vi "newValueStep.vi"(8 "error in (no error)":errorcluster, 11 "RampAction in":refnum<class "RampAction.lvclass">) -> (0 "error out":errorcluster, 3 "RampAction out":refnum<class "RampAction.lvclass">)   [LabVIEW 2009, in "Views.lvlib" / "ScriptEditor.lvlib" / "RampAction.lvclass"]
uses:
  RampAction.lvclass
  RampAction.lvclass/RampAction.ctl
  Tools/Scripting/ScriptingEvent/ScriptEvents/Ramp/RampEvent/RampEvent.lvclass
  ActionPanel.lvclass
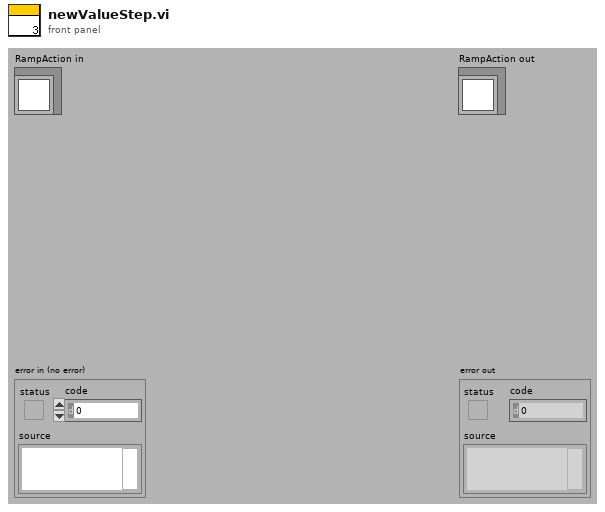
[diagram p1: front panel]
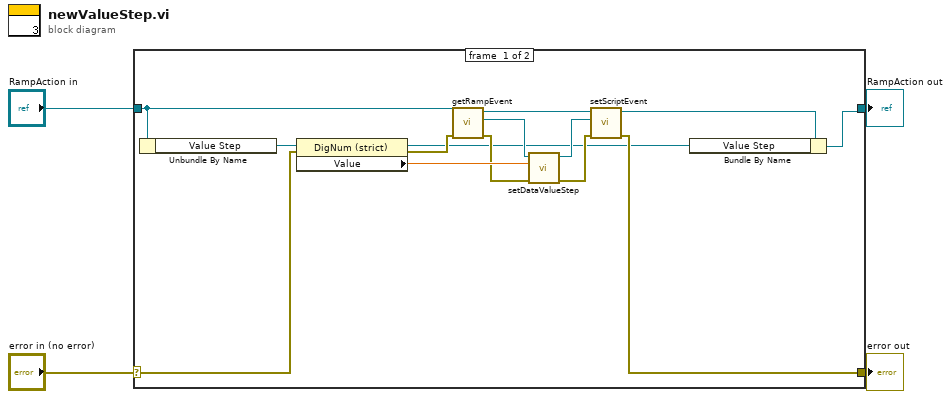
[diagram p0: block diagram]
diagram:
  n1 = case shown="No Error" "error in (no error)" {
    selector: "error in (no error)" -> [w17 w20]
    tunnel: [w8 w20] -> w3
    tunnel: [w5 w19] -> w1
    tunnel: "RampAction in" -> [w16 w19]
    frame #0 {
      n2 = Unbundle By Name(w16) -> ("Value Step"=w18:refnum<vi>)
      n3 = property class="DigNum (strict)"(reference=w18, error in=w17) -> (reference out=w7:refnum<vi>, error out=w15:errorcluster, "Value"=w13:dbl)
      n4 = call "getRampEvent.vi"("error in (no error)"=w15, "RampAction in"=w16) -> ("error out"=w12:errorcluster, "RampEvent"=w14:refnum<class "RampEvent.lvclass">, "RampAction out"=w11:refnum<class "RampAction.lvclass">)  [unwired: 7 in]
      n5 = call "setDataValueStep.vi"("error in (no error)"=w12, "dataValueStep"=w13, "RampEvent.lvclass in"=w14) -> ("error out"=w9:errorcluster, "RampEvent.lvclass out"=w10:refnum<class "RampEvent.lvclass">)  [unwired: 7 in]
      n6 = call "setScriptEvent.vi"("error in (no error)"=w9, "ScriptEvent.lvclass"=w10, "ActionPanel.lvclass in"=w11) -> ("error out"=w8:errorcluster, "ActionPanel.lvclass out"=w6:refnum<class "RampAction.lvclass">)  [unwired: 7 in]
      n7 = Bundle By Name(cluster=w6, "Value Step"=w7) -> (w5:refnum<class "RampAction.lvclass">)
    }
    frame #1 {
    }
  }
  "error out" <- w3
  "RampAction out" <- w1
